vi "Destructor.vi"(8 "error in (no error)":errorcluster, 11 "Solenoid Valve in":refnum<class "Solenoid Valve.lvclass">) -> (0 "error out":errorcluster, 3 "Solenoid Valve out":refnum<class "Solenoid Valve.lvclass">)   [LabVIEW 2011, in "Solenoid Valve.lvclass"]
uses:
  Solenoid Valve.lvclass
  Solenoid Valve.lvclass/Solenoid Valve.ctl
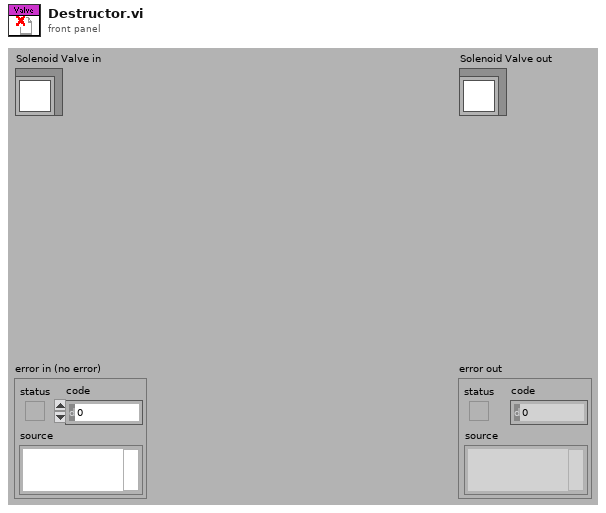
[diagram p1: front panel]
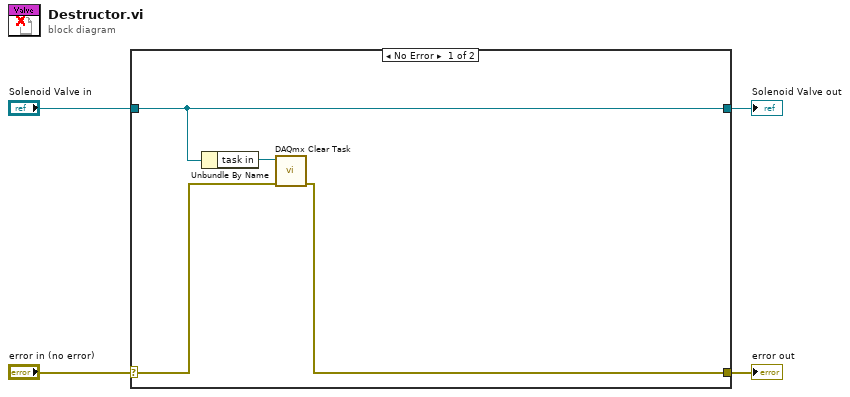
[diagram p0: block diagram]
diagram:
  n1 = case shown="No Error" "error in (no error)" {
    selector: "error in (no error)" -> [w6 w10]
    tunnel: [w5 w10] -> w3
    tunnel: [w8 w9] -> w1
    tunnel: "Solenoid Valve in" -> [w8 w9]
    frame No Error {
      n2 = Unbundle By Name(w8) -> ("task in"=w7:refnum<k21>)
      n3 = call <vilib>:"DAQmx Clear Task.vi"("task in"=w7, "error in"=w6) -> ("error out"=w5:errorcluster)  [unwired: 13 in]
    }
    frame Error {
    }
  }
  "error out" <- w3
  "Solenoid Valve out" <- w1
